vi "EminemCmdShoot.vi"(8 "error in (no error)":errorcluster) -> (0 "error out":errorcluster)   [LabVIEW 2023]
uses:
  <vilib>/Rock Robotics/WPI/ThirdParty/JAS_Junk/TrajLib/Trajectory_Library.lvlib
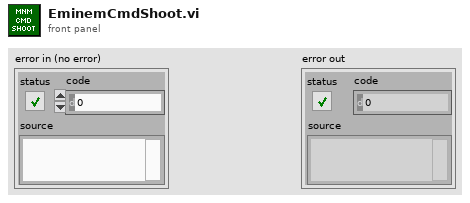
[diagram p1: front panel]
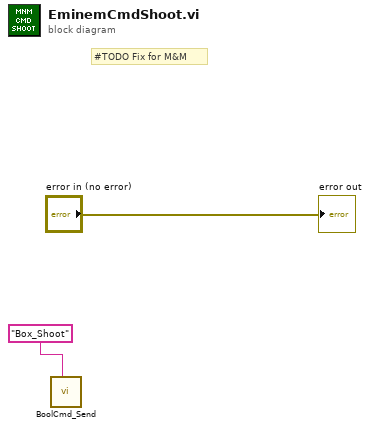
[diagram p0: block diagram]
diagram:
  # "#TODO Fix for M&M"
  n1 = call <vilib>:"BoolCmd_Send.vi"("Command Name"="Box_Shoot") -> ()  [unwired: 10 in, 1 out]
  "error out" <- "error in (no error)"
